vi "Set Component Settings By ID.vi"(8 "error in (no error)":errorcluster, 9 "component settings":T2[](array[typedef]), 10 "settings id":T1={"plugin"=-1, "thread"=-1, "group"=-1, "transfer"=-1, "channel"=-1}, 11 "Framework Configuration in":refnum<class "Framework Configuration.lvclass">) -> (0 "error out":errorcluster, 3 "Framework Configuration out":refnum<class "Framework Configuration.lvclass">)   [LabVIEW 2017, in "DSF Core.lvlib" / "Framework Configuration.lvclass"]
uses:
  Framework Configuration.lvclass
  C:/Git/DSF/Core/Classes/Configuration/Core/Core Configuration.lvclass
  Typedefs/DSF Settings Info.ctl
  Typedefs/DSF Configuration ID.ctl
  Core Configuration.lvclass/Core Configuration.ctl
  Framework Configuration.lvclass/Framework Configuration.ctl
  Plugin/Plugin Configuration.lvclass
  Core Configuration.lvclass
  DSF Core.lvlib
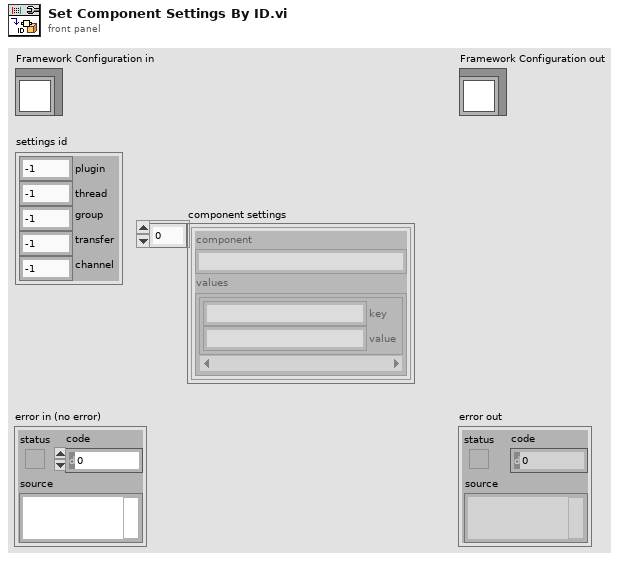
[diagram p1: front panel]
types:
  T1 = typedef "DSF Core.lvlib/DSF Configuration ID.ctl" = cluster{"plugin":i32, "thread":i32, "group":i32, "transfer":i32, "channel":i32}
  T2 = typedef "DSF Core.lvlib/DSF Settings Info.ctl" = cluster{"component":string, "values":cluster{"key":string, "value":string}[]}
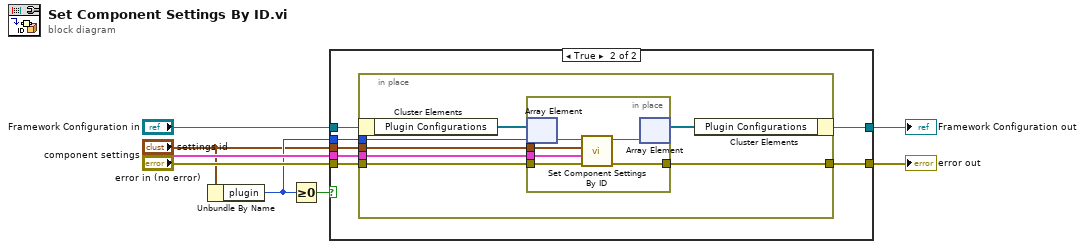
[diagram p0: block diagram]
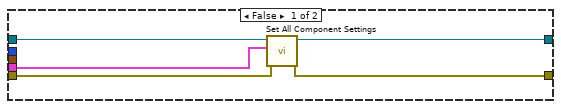
[diagram p2: hidden frame]
diagram:
  n1 = Unbundle By Name("settings id") -> ("plugin"=w3:i32)
  n2 = Greater Or Equal To 0?(x=w3) -> (x >= 0?=w8:bool)
  n3 = case shown="True" w8 {
    tunnel: [w11 w16] -> w2
    tunnel: w3 -> [_ w18]
    tunnel: "error in (no error)" -> [w12 w20]
    tunnel: [w10 w19] -> w6
    tunnel: "settings id" -> [_ w15]
    tunnel: "Framework Configuration in" -> [w13 w17]
    tunnel: "component settings" -> [w9 w14]
    frame False {
      n4 = call "Set All Component Settings.vi"("error in (no error)"=w12, "component settings"=w9, "Runtime Configuration in"=w13) -> ("error out"=w10:errorcluster, "Runtime Configuration out"=w11:refnum<class "Framework Configuration.lvclass">)  [unwired: 7 in]
    }
    frame True {
      n5 = in-place {
        in-place-border: w20 -> [w27]
        in-place-border: [w26] -> w19
        in-place-border: w15 -> [w25]
        in-place-border: w18 -> [w24]
        in-place-border: w14 -> [w21]
        n6 = in-place-cluster #1(w17) -> ("Plugin Configurations"=w23:refnum<class "Plugin Configuration.lvclass">[])
        n7 = in-place {
          in-place-border: w27 -> [w33]
          in-place-border: [w32] -> w26
          in-place-border: w25 -> [w29]
          in-place-border: w21 -> [w28]
          n8 = in-place-array #2(w23, w24) -> (w31:refnum<class "Plugin Configuration.lvclass">)
          n9 = call-dynamic "Set Component Settings By ID.vi"("error in (no error)"=w33, "component settings"=w28, "settings id"=w29, "Plugin Configuration in"=w31) -> ("error out"=w32:errorcluster, "Plugin Configuration out"=w30:refnum<class "Plugin Configuration.lvclass">)  [unwired: 6 in]
          n10 = in-place-array #2(w30) -> (w22:refnum<class "Plugin Configuration.lvclass">[])  [unwired: 1 out]
        }
        n11 = in-place-cluster #1("Plugin Configurations"=w22) -> (w16:refnum<class "Framework Configuration.lvclass">)
      }
    }
  }
  "error out" <- w6
  "Framework Configuration out" <- w2
